vi "Start Logging.vi"(11 "Active Channels":bool[](array[boolean])) -> (0 "error out":errorcluster, 3 "Response":string)   [LabVIEW 2020]
doc: "Starts logging all channels that are set to true in Active Channels input."
uses:
  sub VIs/Globals.vi
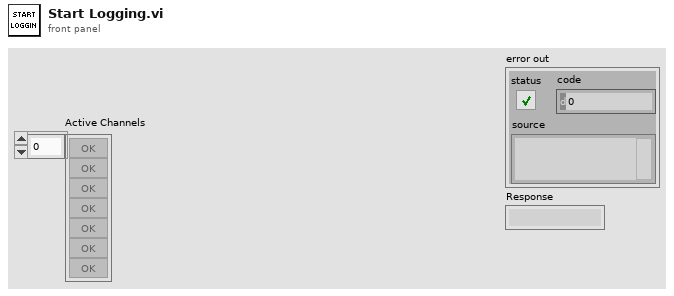
[diagram p1: front panel]
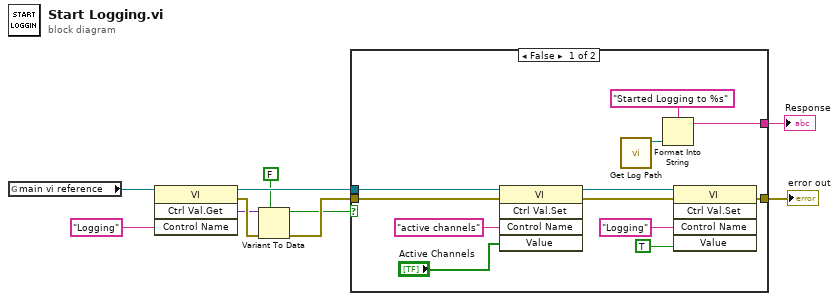
[diagram p0: block diagram]
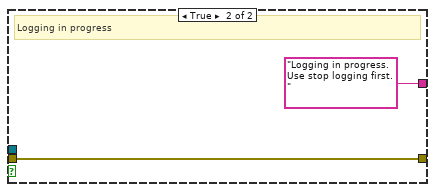
[diagram p2: hidden frame]
diagram:
  n1 = global read "Globals.vi" "main vi reference"() -> (w10:refnum<vi>)
  n2 = invoke class="VI" method="Ctrl Val.Get"(reference=w10, "Control Name"="Logging") -> (reference out=w9:refnum<vi>, error out=w8:errorcluster, "Get Control Value Variant"=w4:variant)  [unwired: 2 in, 1 out]
  n3 = Variant To Data(error in=w8, type=FALSE, Variant=w4) -> (data=w2:bool, error out=w5:errorcluster)
  n4 = case shown="False" w2 {
    tunnel: w9 -> [w17 _]
    tunnel: [w16 w24] -> w7
    tunnel: w5 -> [w15 w24]
    tunnel: [w12 "Logging in progress. Use stop logging first." ("source")] -> w1
    frame False {
      n5 = invoke class="VI" method="Ctrl Val.Set"(reference=w17, error in=w15, "Control Name"="active channels", "Value"="Active Channels") -> (reference out=w11:refnum<vi>, error out=w21:errorcluster)  [unwired: 1 in, 3 out]
      n6 = call "Get Log Path.vi"() -> ("appended path"=w13:path)  [unwired: 11 in]
      n7 = Format Into String(format string="Started Logging to %s" ("Control Name"), w13) -> (resulting string=w12:string)  [unwired: 2 in, 1 out]
      n8 = invoke class="VI" method="Ctrl Val.Set"(reference=w11, error in=w21, "Control Name"="Logging", "Value"=TRUE) -> (error out=w16:errorcluster)  [unwired: 1 in, 4 out]
    }
    frame True {
      # "Logging in progress"
    }
  }
  "error out" <- w7
  "Response" <- w1
